vi "prac5_2.vi"() -> ()   [LabVIEW 2026]
panel:
  out "Array":i32[](array[numeric])
  in  "Numeric":dbl
  in  "DOWN":bool
  out "Boolean 2":bool
  in  "UP":bool
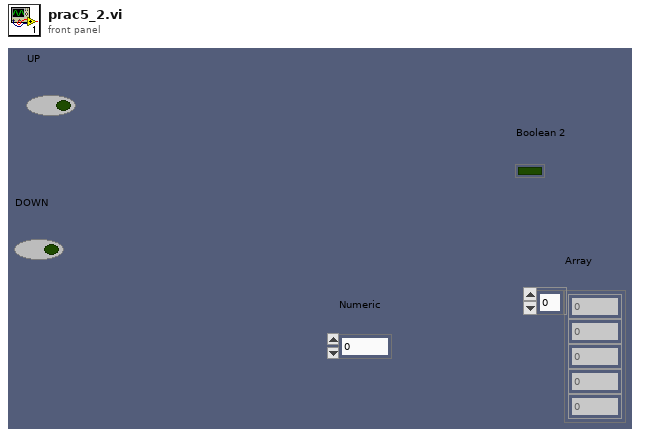
[diagram p1: front panel]
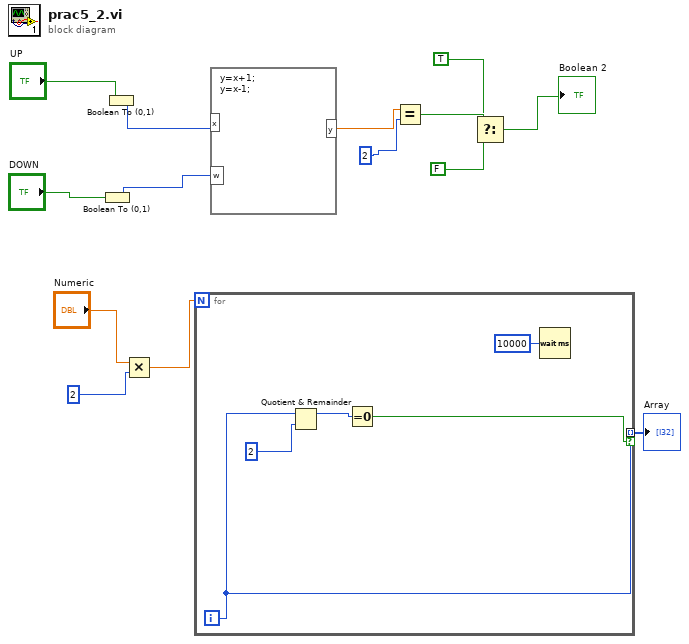
[diagram p0: block diagram]
diagram:
  n1 = Boolean To (0,1)(Boolean="DOWN") -> (0, 1=w5:i16)
  n2 = Boolean To (0,1)(Boolean="UP") -> (0, 1=w14:i16)
  n3 = Multiply(x="Numeric", y=2) -> (x*y=w2:dbl)
  n4 = for {
    N: w2 -> [_]
    tunnel: [w17] -> w1 mode=indexing if=w16
    i -> [w17]
    n5 = Quotient & Remainder(x=w17, y=2) -> (x-y*floor(x/y)=w18:i32)  [unwired: 1 out]
    n6 = Equal To 0?(x=w18) -> (x = 0?=w16:bool)
    n7 = Wait (ms)(milliseconds to wait=u32 10000) -> ()  [unwired: 1 out]
  }
  "Array" <- w1
  n8 = formula code="y=x+1;\ny=x-1;"("x"=w14, "w"=w5) -> ("y"=w13:dbl)
  n9 = Equal?(x=w13, y=2) -> (x = y?=w12:bool)
  n10 = Select(t=TRUE, s=w12, f=FALSE) -> (s? t:f=→"Boolean 2":bool)
